vi "PlotSwerve.vi"(10 "Pod Plot Data In":T1(array[cluster]), 11 "Picture refrence":refnum<vi>) -> ()   [LabVIEW 2014]
panel:
  out "Scalar":dbl
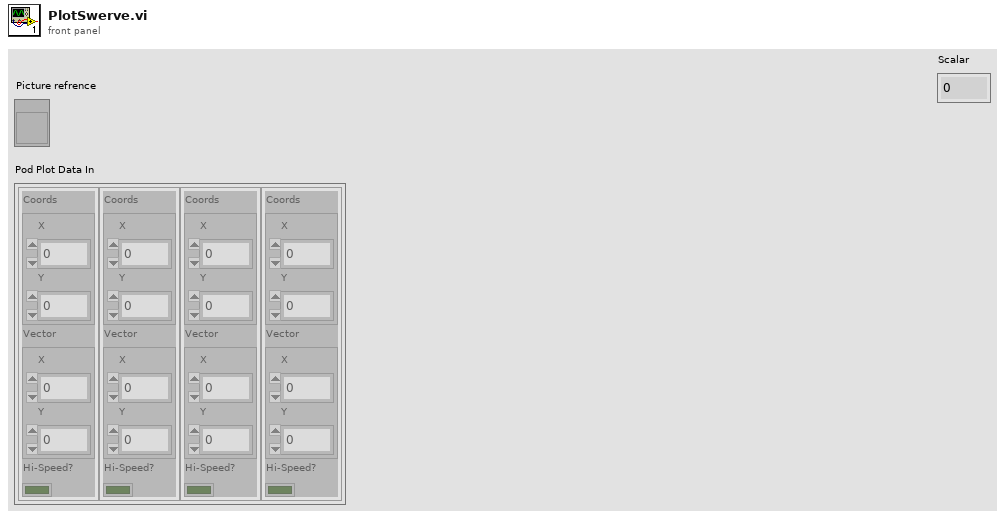
[diagram p1: front panel]
types:
  T1 = cluster{"Coords":cluster{"X":dbl, "Y":dbl}, "Vector":cluster{"X":dbl, "Y":dbl}, "Hi-Speed?":bool}[]
  T2 = cluster{"Y":cluster{"Max":dbl, "Min":dbl}, "X":cluster{"Max":dbl, "Min":dbl}}
  T3 = cluster{"Coords":cluster{"X":dbl, "Y":dbl}, "Vector":cluster{"X":dbl, "Y":dbl}}
  T4 = typedef "LVBoundsTypeDef.ctl" = cluster{"Width":u32, "Height":u32}
  T5 = cluster{"Coords":cluster{"X":dbl, "Y":dbl}, "Vector":cluster{"X":dbl, "Y":dbl}}[]
  T6 = cluster{"Width":u16, "Style":enum32{"Solid", "Dash", "Dot", "DashDot", "DashDotDot"}}
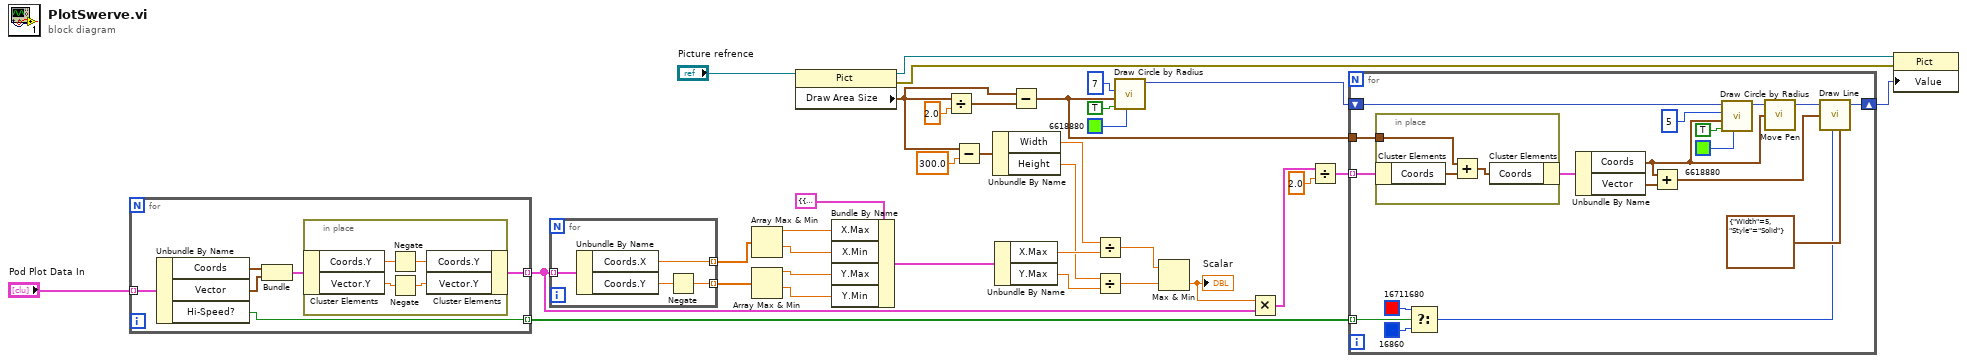
[diagram p0: block diagram]
diagram:
  n1 = for {
    tunnel: "Pod Plot Data In" -> [w40] mode=indexing
    tunnel: [w41] -> w3 mode=indexing
    tunnel: [w36] -> w1 mode=indexing
    n2 = Unbundle By Name(w40) -> ("Coords"=w39:cluster{"X":dbl, "Y":dbl}, "Vector"=w38:cluster{"X":dbl, "Y":dbl}, "Hi-Speed?"=w36:bool)
    n3 = Bundle("Coords"=w39, "Vector"=w38) -> (w37:T3)  [unwired: 1 in]
    n4 = in-place {
      n5 = in-place-cluster #1(w37) -> ("Coords.Y"=w45:dbl, "Vector.Y"=w43:dbl)
      n6 = Negate(x=w45) -> (-x=w44:dbl)
      n7 = Negate(x=w43) -> (-x=w42:dbl)
      n8 = in-place-cluster #1("Coords.Y"=w44, "Vector.Y"=w42) -> (w41:T3)
    }
  }
  n9 = for {
    tunnel: w3 -> [w49] mode=indexing
    tunnel: [w48] -> w33 mode=indexing
    tunnel: [w46] -> w34 mode=indexing
    n10 = Unbundle By Name(w49) -> ("Coords.X"=w48:dbl, "Coords.Y"=w47:dbl)
    n11 = Negate(x=w47) -> (-x=w46:dbl)
  }
  n12 = Array Max & Min(array=w33) -> (max value=w31:dbl, min value=w30:dbl)  [unwired: 2 out]
  n13 = Array Max & Min(array=w34) -> (max value=w29:dbl, min value=w28:dbl)  [unwired: 2 out]
  n14 = property class="Pict"(reference="Picture refrence") -> (reference out=w10:refnum<vi>, error out=w9:errorcluster, "Draw Area Size"=w16:T4)  [unwired: 1 in]
  n15 = Bundle By Name(cluster=T2 {"Y"={"Max"=0.0, "Min"=0.0}, "X"={"Max"=0.0, "Min"=0.0}}, "X.Max"=w31, "X.Min"=w30, "Y.Max"=w29, "Y.Min"=w28) -> (w25:T2)
  n16 = Divide(x=w16, y=2.0) -> (x/y=w17:cluster{"Width":dbl, "Height":dbl})
  n17 = Subtract(x=w16, y=300.0) -> (x-y=w26:cluster{"Width":dbl, "Height":dbl})
  n18 = Unbundle By Name(w26) -> ("Width"=w24:dbl, "Height"=w21:dbl)
  n19 = Unbundle By Name(w25) -> ("X.Max"=w23:dbl, "Y.Max"=w22:dbl)
  n20 = Subtract(x=w16, y=w17) -> (x-y=w15:cluster{"Width":dbl, "Height":dbl})
  n21 = Divide(x=w24, y=w23) -> (x/y=w19:dbl)
  n22 = Divide(x=w21, y=w22) -> (x/y=w20:dbl)
  n23 = call <vilib>:"Draw Circle by Radius.vi"("color(black)"=u32 6618880, "fill?(F)"=TRUE, "pixel center"=w15, "radius"=i16 7) -> ("new picture"=w11:picture)  [unwired: 7 in]
  n24 = Max & Min(x=w19, y=w20) -> (min(x,y)=w7:dbl)  [unwired: 1 out]
  "Scalar" <- w7
  n25 = Multiply(x=w7, y=w3) -> (x*y=w6:T5)
  n26 = Divide(x=w6, y=2.0 ("scl")) -> (x/y=w5:T5)
  n27 = for {
    tunnel: w5 -> [w67] mode=indexing
    tunnel: w15 -> [w66]
    shift-right: [w58] -> w8
    shift-left: w11 -> [w64]
    tunnel: w1 -> [w50] mode=indexing
    n28 = in-place {
      in-place-border: w66 -> [w68]
      n29 = in-place-cluster #2(w67) -> ("Coords"=w70:cluster{"X":dbl, "Y":dbl})
      n30 = Add(x=w68, y=w70) -> (x+y=w69:cluster{dbl, dbl})
      n31 = in-place-cluster #2("Coords"=w69) -> (w65:T3)
    }
    n32 = Select(t=u32 16711680 ("color(black)"), s=w50, f=u32 16860 ("color(black)")) -> (s? t:f=w52:u32)
    n33 = Unbundle By Name(w65) -> ("Coords"=w56:cluster{"X":dbl, "Y":dbl}, "Vector"=w55:cluster{"X":dbl, "Y":dbl})
    n34 = Add(x=w56, y=w55) -> (x+y=w54:cluster{"X":dbl, "Y":dbl})
    n35 = call <vilib>:"Draw Circle by Radius.vi"("color(black)"=u32 6618880, "fill?(F)"=TRUE, "pixel center"=w56, "radius"=i16 5, "picture"=w64) -> ("new picture"=w60:picture)  [unwired: 6 in]
    n36 = call <vilib>:"Move Pen.vi"("new position"=w56, "picture"=w60) -> ("new picture"=w59:picture)  [unwired: 3 in]
    n37 = call <vilib>:"Draw Line.vi"("picture"=w59, "end point"=w54, "color(black)"=w52, "pen"=T6 {"Width"=5, "Style"=enum."Solid"}) -> ("new picture"=w58:picture)  [unwired: 5 in]
  }
  n38 = property class="Pict"(reference=w10, error in=w9, "Value"=w8) -> ()  [unwired: 2 out]
